vi "Two Ball Hot.vi"() -> ()   [LabVIEW 2014]
uses:
  Team Code/Robot Global Data.vi
panel:
  out "Left Triggered":bool
  in  "Turn Angle":dbl=-13.0
  out "Angle":dbl
  out "Distance (in)":dbl
  in  "Min. Power":dbl=0.1 format="%#_13g"
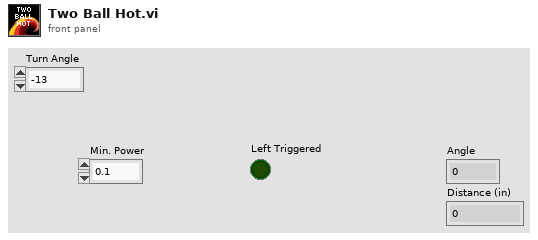
[diagram p1: front panel]
types:
  T1 = cluster{"FIRE!!!":bool, "Loader":bool, "Lock":bool, "Load":bool, "Pass":bool, "Grab":bool, "PANIC":bool, "Don't Cock":bool, "Roller Speed":dbl}
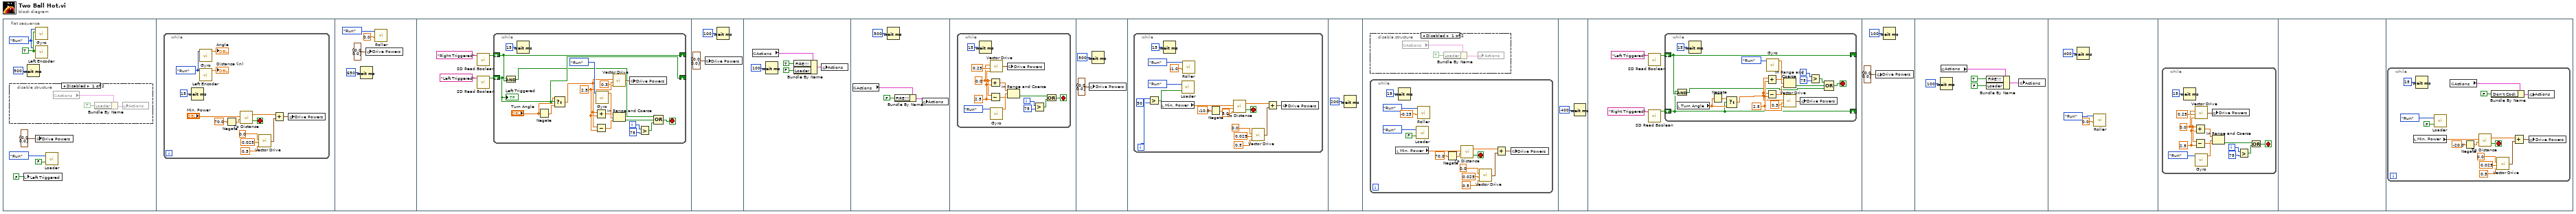
[diagram p0: block diagram]
diagram:
  n1 = flat-sequence {
    frame #0 {
      w6 = enum16{"Start", "Run", "End"}."Run" ("Enum")
      w7 = TRUE ("Reset")
      n2 = disable-structure shown="Disabled" {
        frame Disabled {
          n3 = global read "Robot Global Data.vi" "Actions"() -> (w9:T1)
          n4 = Bundle By Name(cluster=w9, "Loader"=TRUE ("Primary Action")) -> (w10:T1)
          n5 = global write "Robot Global Data.vi" "Actions"(w10) -> ()
        }
        frame Enabled {
        }
      }
      n6 = local write "Left Triggered"(FALSE ("Left Triggered")) -> ()
      n7 = Wait (ms)(milliseconds to wait=u32 500) -> ()  [unwired: 1 out]
      n8 = call "Gyro.vi"("Reset"=w7, "Enum"=w6) -> ()  [unwired: 9 in, 1 out]
      n9 = call "Left Encoder.vi"("Reset"=w7, "Enum"=w6) -> ()  [unwired: 8 in, 2 out]
      n10 = global write "Robot Global Data.vi" "Drive Powers"(cluster{"Right":dbl, "Left":dbl} {"Right"=0.0, "Left"=0.0} ("Drive Powers")) -> ()
      n11 = call "Loader.vi"("Down (Forward)"=FALSE, "Enum"=enum16{"Start", "Run", "End"}."Run") -> ()  [unwired: 1 out]
    }
    frame #1 {
      n12 = while {
        stop <- w23 stop-if-true
        w16 = enum16{"Start", "Run", "End"}."Run" ("Enum")
        n13 = Wait (ms)(milliseconds to wait=u32 15) -> ()  [unwired: 1 out]
        n14 = call "Gyro.vi"("Enum"=w16) -> ("Angle"=→"Angle":dbl)  [unwired: 10 in]
        n15 = call "Left Encoder.vi"("Enum"=w16) -> ("Distance (in)"=→"Distance (in)":dbl)  [unwired: 9 in, 1 out]
        n16 = Negate(x=70.0) -> (-x=w14:dbl)
        n17 = call "To Distance.vi"("Destination Dist (in)"=w14, "Min. Power"="Min. Power") -> ("Reached Distance"=w23:bool, "Base Speed"=w13:dbl)  [unwired: 2 in]
        n18 = call "Vector Drive.vi"("Tolerance"=0.5, "Min. Power"=0.025, "Angle"=0.0) -> ("Motor Powers"=w19:cluster{"RMotor":dbl, "LMotor":dbl})  [unwired: 1 in]
        n19 = Add(x=w13, y=w19) -> (x+y=w18:cluster{"RMotor":dbl, "LMotor":dbl})
        n20 = global write "Robot Global Data.vi" "Drive Powers"(w18) -> ()
      }
    }
    frame #2 {
      n21 = Wait (ms)(milliseconds to wait=u32 650) -> ()  [unwired: 1 out]
      n22 = global write "Robot Global Data.vi" "Drive Powers"(cluster{"Right":dbl, "Left":dbl} {"Right"=0.0, "Left"=0.0} ("Drive Powers")) -> ()
      n23 = call "Roller.vi"("Power"=0.0, "Enum"=enum16{"Start", "Run", "End"}."Run") -> ()  [unwired: 2 in]
    }
    frame #3 {
      n24 = call <vilib>:"SD Read Boolean.vi"("Name"="Right Triggered") -> ("Boolean"=w29:bool)  [unwired: 8 in, 2 out]
      n25 = call <vilib>:"SD Read Boolean.vi"("Name"="Left Triggered") -> ("Boolean"=w31:bool)  [unwired: 8 in, 2 out]
      n26 = while {
        shift-right: [w37] -> _
        shift-left: w31 -> [w37]
        shift-right: [w38] -> _
        shift-left: w29 -> [w38]
        i -> [w43]
        stop <- w39 stop-if-true
        w44 = 2.5 ("Tolerance")
        n27 = And(x=w37, y=w38) -> (x .and. y?=w34:bool)
        n28 = Wait (ms)(milliseconds to wait=u32 15) -> ()  [unwired: 1 out]
        n29 = Negate(x="Turn Angle") -> (-x=w36:dbl)
        n30 = Select(t="Turn Angle", s=w37, f=w36) -> (s? t:f=w33:dbl)
        n31 = Add(x=w33, y=w44) -> (x+y=w46:dbl)
        n32 = Subtract(x=w33, y=w44) -> (x-y=w45:dbl)
        n33 = call "Gyro.vi"("Enum"=enum16{"Start", "Run", "End"}."Run") -> ("Angle"=w48:dbl)  [unwired: 10 in]
        n34 = call "Vector Drive.vi"("Tolerance"=w44, "Min. Power"=0.3, "Angle"=w33) -> ("Motor Powers"=w49:cluster{"RMotor":dbl, "LMotor":dbl})  [unwired: 1 in]
        n35 = In Range and Coerce(upper limit=w46, x=w48, lower limit=w45) -> (In Range?=w41:bool)  [unwired: 1 out]
        n36 = global write "Robot Global Data.vi" "Drive Powers"(w49) -> ()
        n37 = Greater?(x=w43, y=75) -> (0:w40:bool)
        n38 = Compound Arithmetic op=OR(w34, w41, w40) -> (w39:bool)
        "Left Triggered" <- w37
      }
    }
    frame #4 {
      n39 = global write "Robot Global Data.vi" "Drive Powers"(cluster{"Right":dbl, "Left":dbl} {"Right"=0.0, "Left"=0.0} ("Drive Powers")) -> ()
      n40 = Wait (ms)(milliseconds to wait=u32 100) -> ()  [unwired: 1 out]
    }
    frame #5 {
      n41 = global read "Robot Global Data.vi" "Actions"() -> (w57:T1)
      n42 = Wait (ms)(milliseconds to wait=u32 100) -> ()  [unwired: 1 out]
      n43 = Bundle By Name(cluster=w57, "FIRE!!!"=TRUE ("Primary Action"), "Loader"=FALSE) -> (w58:T1)
      n44 = global write "Robot Global Data.vi" "Actions"(w58) -> ()
    }
    frame #6 {
      n45 = global read "Robot Global Data.vi" "Actions"() -> (w60:T1)
      n46 = Wait (ms)(milliseconds to wait=u32 500) -> ()  [unwired: 1 out]
      n47 = Bundle By Name(cluster=w60, "FIRE!!!"=FALSE ("Primary Action")) -> (w59:T1)
      n48 = global write "Robot Global Data.vi" "Actions"(w59) -> ()
    }
    frame #7 {
      n49 = while {
        i -> [w67]
        stop <- w65 stop-if-true
        w68 = 0.0 ("Tolerance")
        w69 = 2.5 ("Tolerance")
        n50 = Wait (ms)(milliseconds to wait=u32 15) -> ()  [unwired: 1 out]
        n51 = Add(x=w68, y=w69) -> (x+y=w71:dbl)
        n52 = Subtract(x=w68, y=w69) -> (x-y=w70:dbl)
        n53 = call "Vector Drive.vi"("Tolerance"=w69, "Min. Power"=0.25, "Angle"=w68) -> ("Motor Powers"=w74:cluster{"RMotor":dbl, "LMotor":dbl})  [unwired: 1 in]
        n54 = call "Gyro.vi"("Enum"=enum16{"Start", "Run", "End"}."Run") -> ("Angle"=w73:dbl)  [unwired: 10 in]
        n55 = global write "Robot Global Data.vi" "Drive Powers"(w74) -> ()
        n56 = In Range and Coerce(upper limit=w71, x=w73, lower limit=w70) -> (In Range?=w64:bool)  [unwired: 1 out]
        n57 = Greater?(x=w67, y=75) -> (0:w63:bool)
        n58 = Or(x=w64, y=w63) -> (x .or. y?=w65:bool)
      }
    }
    frame #8 {
      n59 = global write "Robot Global Data.vi" "Drive Powers"(cluster{"Right":dbl, "Left":dbl} {"Right"=0.0, "Left"=0.0} ("Drive Powers")) -> ()
      n60 = Wait (ms)(milliseconds to wait=u32 500) -> ()  [unwired: 1 out]
    }
    frame #9 {
      n61 = while {
        i -> [w81]
        stop <- w96 stop-if-true
        n62 = Greater?(x=w81, y=50) -> (0:w79:bool)
        n63 = local read "Min. Power"() -> (w84:dbl)
        n64 = Wait (ms)(milliseconds to wait=u32 15) -> ()  [unwired: 1 out]
        n65 = call "Loader.vi"("Down (Forward)"=w79, "Enum"=enum16{"Start", "Run", "End"}."Run") -> ()  [unwired: 1 out]
        n66 = call "Roller.vi"("Power"=-1.0, "Enum"=enum16{"Start", "Run", "End"}."Run") -> ()  [unwired: 2 in]
        n67 = Negate(x=-10.0) -> (-x=w90:dbl)
        n68 = call "To Distance.vi"("Tolerance"=5.0, "Destination Dist (in)"=w90, "Min. Power"=w84) -> ("Reached Distance"=w96:bool, "Base Speed"=w88:dbl)  [unwired: 1 in]
        n69 = call "Vector Drive.vi"("Tolerance"=0.5, "Min. Power"=0.025, "Angle"=0.0) -> ("Motor Powers"=w92:cluster{"RMotor":dbl, "LMotor":dbl})  [unwired: 1 in]
        n70 = Add(x=w88, y=w92) -> (x+y=w91:cluster{"RMotor":dbl, "LMotor":dbl})
        n71 = global write "Robot Global Data.vi" "Drive Powers"(w91) -> ()
      }
    }
    frame #10 {
      n72 = Wait (ms)(milliseconds to wait=u32 200) -> ()  [unwired: 1 out]
    }
    frame #11 {
      n73 = disable-structure shown="Disabled" {
        frame Disabled {
          n74 = global read "Robot Global Data.vi" "Actions"() -> (w99:T1)
          n75 = Bundle By Name(cluster=w99, "Loader"=TRUE) -> (w98:T1)
          n76 = global write "Robot Global Data.vi" "Actions"(w98) -> ()
        }
        frame Enabled {
        }
      }
      n77 = while {
        stop <- w115 stop-if-true
        n78 = local read "Min. Power"() -> (w104:dbl)
        n79 = Wait (ms)(milliseconds to wait=u32 15) -> ()  [unwired: 1 out]
        n80 = call "Loader.vi"("Down (Forward)"=FALSE, "Enum"=enum16{"Start", "Run", "End"}."Run") -> ()  [unwired: 1 out]
        n81 = call "Roller.vi"("Power"=-0.25, "Enum"=enum16{"Start", "Run", "End"}."Run") -> ()  [unwired: 2 in]
        n82 = Negate(x=70.0) -> (-x=w109:dbl)
        n83 = call "To Distance.vi"("Destination Dist (in)"=w109, "Min. Power"=w104) -> ("Reached Distance"=w115:bool, "Base Speed"=w107:dbl)  [unwired: 2 in]
        n84 = call "Vector Drive.vi"("Tolerance"=0.5, "Min. Power"=0.025, "Angle"=0.0) -> ("Motor Powers"=w111:cluster{"RMotor":dbl, "LMotor":dbl})  [unwired: 1 in]
        n85 = Add(x=w107, y=w111) -> (x+y=w110:cluster{"RMotor":dbl, "LMotor":dbl})
        n86 = global write "Robot Global Data.vi" "Drive Powers"(w110) -> ()
      }
    }
    frame #12 {
      n87 = Wait (ms)(milliseconds to wait=u32 400) -> ()  [unwired: 1 out]
    }
    frame #13 {
      n88 = call <vilib>:"SD Read Boolean.vi"("Name"="Left Triggered") -> ("Boolean"=w117:bool)  [unwired: 8 in, 2 out]
      n89 = call <vilib>:"SD Read Boolean.vi"("Name"="Right Triggered") -> ("Boolean"=w118:bool)  [unwired: 8 in, 2 out]
      n90 = while {
        shift-right: [w123] -> _
        shift-left: w118 -> [w123]
        shift-right: [w124] -> _
        shift-left: w117 -> [w124]
        i -> [w126]
        stop <- w129 stop-if-true
        w132 = 2.5 ("Tolerance")
        n91 = And(x=w123, y=w124) -> (x .and. y?=w121:bool)
        n92 = local read "Turn Angle"() -> (w130:dbl)
        n93 = Wait (ms)(milliseconds to wait=u32 15) -> ()  [unwired: 1 out]
        n94 = Negate(x=w130) -> (-x=w131:dbl)
        n95 = Select(t=w131, s=w123, f=w130) -> (s? t:f=w122:dbl)
        n96 = Add(x=w122, y=w132) -> (x+y=w134:dbl)
        n97 = Subtract(x=w122, y=w132) -> (x-y=w133:dbl)
        n98 = call "Gyro.vi"("Enum"=enum16{"Start", "Run", "End"}."Run") -> ("Angle"=w136:dbl)  [unwired: 10 in]
        n99 = In Range and Coerce(upper limit=w134, x=w136, lower limit=w133) -> (In Range?=w128:bool)  [unwired: 1 out]
        n100 = call "Vector Drive.vi"("Tolerance"=w132, "Min. Power"=0.3, "Angle"=w122) -> ("Motor Powers"=w137:cluster{"RMotor":dbl, "LMotor":dbl})  [unwired: 1 in]
        n101 = global write "Robot Global Data.vi" "Drive Powers"(w137) -> ()
        n102 = Greater?(x=w126, y=75) -> (0:w127:bool)
        n103 = Compound Arithmetic op=OR(w127, w128, w121) -> (w129:bool)
      }
    }
    frame #14 {
      n104 = global write "Robot Global Data.vi" "Drive Powers"(cluster{"Right":dbl, "Left":dbl} {"Right"=0.0, "Left"=0.0} ("Drive Powers")) -> ()
      n105 = Wait (ms)(milliseconds to wait=u32 100) -> ()  [unwired: 1 out]
    }
    frame #15 {
      n106 = Wait (ms)(milliseconds to wait=u32 100) -> ()  [unwired: 1 out]
      n107 = global read "Robot Global Data.vi" "Actions"() -> (w146:T1)
      n108 = Bundle By Name(cluster=w146, "FIRE!!!"=TRUE ("Primary Action"), "Loader"=FALSE) -> (w145:T1)
      n109 = global write "Robot Global Data.vi" "Actions"(w145) -> ()
    }
    frame #16 {
      n110 = Wait (ms)(milliseconds to wait=u32 400) -> ()  [unwired: 1 out]
      n111 = call "Roller.vi"("Power"=0.0, "Enum"=enum16{"Start", "Run", "End"}."Run") -> ()  [unwired: 2 in]
    }
    frame #17 {
      n112 = while {
        i -> [w154]
        stop <- w152 stop-if-true
        w155 = 0.0 ("Tolerance")
        w156 = 2.5 ("Tolerance")
        n113 = Wait (ms)(milliseconds to wait=u32 15) -> ()  [unwired: 1 out]
        n114 = Add(x=w155, y=w156) -> (x+y=w158:dbl)
        n115 = Subtract(x=w155, y=w156) -> (x-y=w157:dbl)
        n116 = call "Vector Drive.vi"("Tolerance"=w156, "Min. Power"=0.25, "Angle"=w155) -> ("Motor Powers"=w161:cluster{"RMotor":dbl, "LMotor":dbl})  [unwired: 1 in]
        n117 = call "Gyro.vi"("Enum"=enum16{"Start", "Run", "End"}."Run") -> ("Angle"=w160:dbl)  [unwired: 10 in]
        n118 = global write "Robot Global Data.vi" "Drive Powers"(w161) -> ()
        n119 = In Range and Coerce(upper limit=w158, x=w160, lower limit=w157) -> (In Range?=w151:bool)  [unwired: 1 out]
        n120 = Greater?(x=w154, y=75) -> (0:w150:bool)
        n121 = Or(x=w151, y=w150) -> (x .or. y?=w152:bool)
      }
    }
    frame #18 {
    }
    frame #19 {
      n122 = while {
        stop <- w179 stop-if-true
        n123 = local read "Min. Power"() -> (w169:dbl)
        n124 = Wait (ms)(milliseconds to wait=u32 15) -> ()  [unwired: 1 out]
        n125 = call "Loader.vi"("Down (Forward)"=FALSE, "Enum"=enum16{"Start", "Run", "End"}."Run") -> ()  [unwired: 1 out]
        n126 = global read "Robot Global Data.vi" "Actions"() -> (w166:T1)
        n127 = Negate(x=-20.0) -> (-x=w173:dbl)
        n128 = call "To Distance.vi"("Destination Dist (in)"=w173, "Min. Power"=w169) -> ("Reached Distance"=w179:bool, "Base Speed"=w172:dbl)  [unwired: 2 in]
        n129 = Bundle By Name(cluster=w166, "Don't Cock"=FALSE ("Primary Action")) -> (w165:T1)
        n130 = call "Vector Drive.vi"("Tolerance"=0.5, "Min. Power"=0.025, "Angle"=0.0) -> ("Motor Powers"=w175:cluster{"RMotor":dbl, "LMotor":dbl})  [unwired: 1 in]
        n131 = Add(x=w172, y=w175) -> (x+y=w174:cluster{"RMotor":dbl, "LMotor":dbl})
        n132 = global write "Robot Global Data.vi" "Actions"(w165) -> ()
        n133 = global write "Robot Global Data.vi" "Drive Powers"(w174) -> ()
      }
    }
  }
